vi "XY_Dialog.vi"(1 "Y输入":dbl[][](array[numeric]), 2 "X输入":dbl[][](array[numeric])) -> ()   [LabVIEW 2020]
panel:
  out "XY Graph":cluster{"Y":dbl[], "Y":dbl[]}[](graph) caption="曲线图"
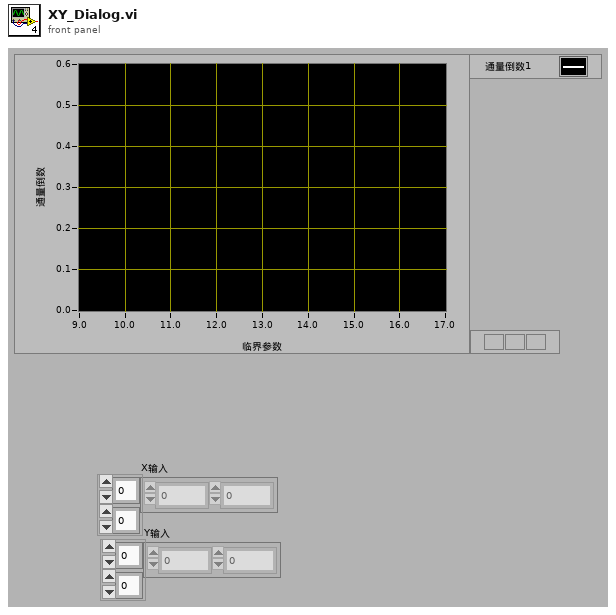
[diagram p1: front panel]
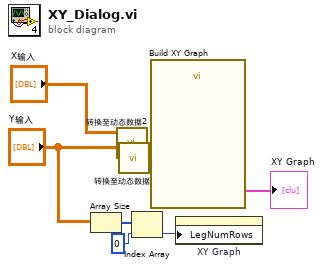
[diagram p0: block diagram]
diagram:
  n1 = Array Size(array="Y输入") -> (size(s)=w3:i32[])
  n2 = call "转换至动态数据2"("2D Array"="X输入") -> ("Dynamic Data Type"=w6:dynamicdata)  [unwired: 3 in]
  n3 = call "转换至动态数据"("2D Array"="Y输入") -> ("Dynamic Data Type"=w7:dynamicdata)  [unwired: 3 in]
  n4 = Index Array(array=w3, index=0 ("索引")) -> (element=w1:i32)
  n5 = call "Build XY Graph"("Y Input"=w7, "X Input"=w6) -> ("XY Graph"=→"XY Graph":cluster{"Y":dbl[], "Y":dbl[]}[])  [unwired: 3 in, 6 out]
  n6 = property on="XY Graph" class="XYGraph (strict)"("LegNumRows"=w1) -> ()  [unwired: 2 in, 2 out]
